vi "Initialize.vi"(8 "error in (no error)":errorcluster, 10 "Numeric":dbl) -> (0 "error out":errorcluster, 3 "Class Alpha out":refnum<class "Class Alpha.lvclass">)   [LabVIEW 2023, in "Class Alpha.lvclass"]
doc: "Initialize a Class Alpha object."
uses:
  Class Alpha.lvclass
  Class Alpha.lvclass/Class Alpha.ctl
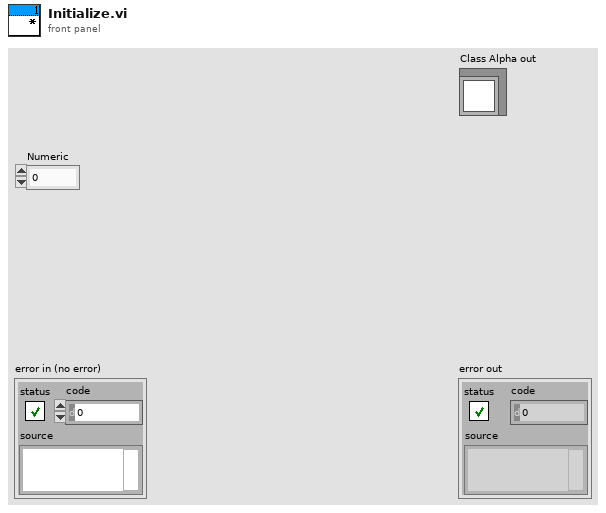
[diagram p1: front panel]
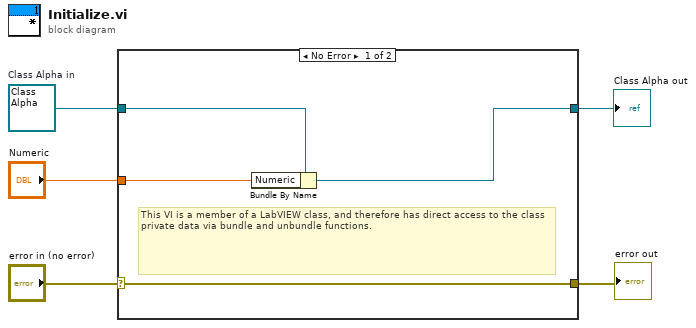
[diagram p0: block diagram]
diagram:
  w3 = refnum<class "Class Alpha.lvclass"> refnum  # Class Alpha in
  n1 = case shown="No Error" "error in (no error)" {
    selector: "error in (no error)" -> [w9 w11]
    tunnel: [w9 w11] -> w4
    tunnel: [w6 w10] -> w2
    tunnel: w3 -> [w8 w10]
    tunnel: "Numeric" -> [w7 _]
    frame No Error {
      # "This VI is a member of a LabVIEW class, and therefore has direct access to the class private data via bundle and unbundle functions."
      n2 = Bundle By Name(cluster=w8, "Numeric"=w7) -> (w6:refnum<class "Class Alpha.lvclass">)
    }
    frame Error {
    }
  }
  "error out" <- w4
  "Class Alpha out" <- w2
